vi "PWM输出.vi"(10 "步骤次数输入":u16, 11 "簇":T1={"工位1"=refnum, "1-3参数设置"=refnum, "总时间"=0, "NG？"=FALSE, "循环次数"=0, "步骤次数"=0, "单个时间"=0, "完成?"=FALSE, "路径"=path "", "1"=0, "2"=0, "3"=0, "4"=0, "AI"=0, "范围"=0, "保存间隔时间"=1} {"保存间隔时间" min=1 step=1}) -> (3 "步骤次数输出":dbl)   [LabVIEW 2012]
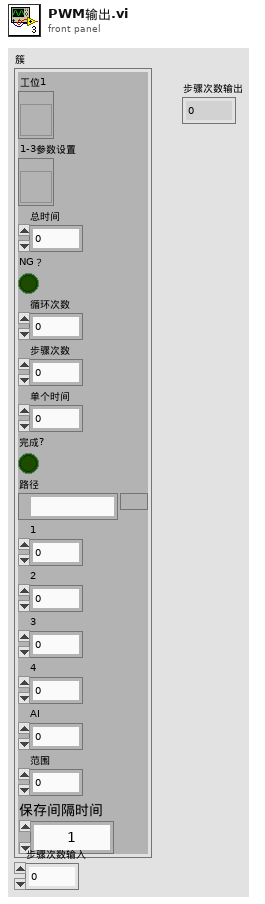
[diagram p1: front panel]
types:
  T1 = typedef "控件 4.ctl" = cluster{"工位1":refnum<vi>, "1-3参数设置":refnum<vi>, "总时间":u32, "NG？":bool, "循环次数":i32, "步骤次数":i32, "单个时间":u32, "完成?":bool, "路径":path, "1":i32, "2":i32, "3":i32, "4":i32, "AI":i32, "范围":i32, "保存间隔时间":u64}
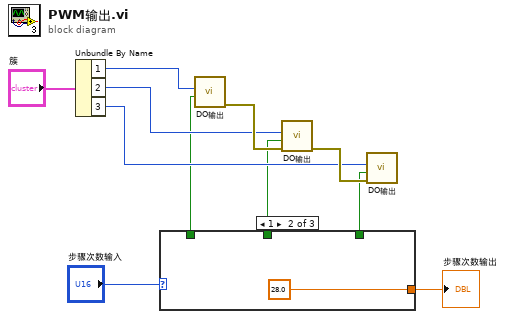
[diagram p0: block diagram]
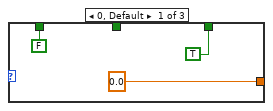
[diagram p2: hidden frame]
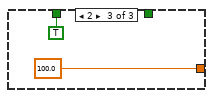
[diagram p3: hidden frame]
diagram:
  n1 = Unbundle By Name("簇") -> ("1"=w6:i32, "2"=w5:i32, "3"=w4:i32)
  n2 = case shown="1" "步骤次数输入" {
    tunnel: [0.0 ("步骤次数") 28.0 ("步骤次数") 100.0 ("步骤次数")] -> w11
    tunnel: [TRUE _ _] -> w3
    tunnel: [_ _ TRUE] -> w2
    tunnel: [FALSE _ _] -> w1
    frame 0, Default {
    }
    frame 1 {
    }
    frame 2 {
    }
  }
  "步骤次数输出" <- w11
  n3 = call "DO输出.vi"("TF"=w1, "序号"=w6) -> ("错误输出"=w8:errorcluster)  [unwired: 9 in]
  n4 = call "DO输出.vi"("错误输入（无错误）"=w8, "TF"=w2, "序号"=w5) -> ("错误输出"=w7:errorcluster)  [unwired: 8 in]
  n5 = call "DO输出.vi"("错误输入（无错误）"=w7, "TF"=w3, "序号"=w4) -> ()  [unwired: 8 in, 1 out]
